vi "DataWriteTxt.vi"(0 "DataFileRef":refnum<file>, 9 "NewDataIn":dbl[](array[numeric]) format="%#_16g", 11 "error in (no error)":errorcluster) -> (4 "DataFileRef Out":refnum<file>, 10 "NewDataOut":dbl[](array[numeric]) format="%#_16g", 15 "error out":errorcluster)   [LabVIEW 2019]
doc: "Ce VI sauvegarde les données d'acquisition pour en garder une copie de sécurité qui peut être rappeller en cas de panne."
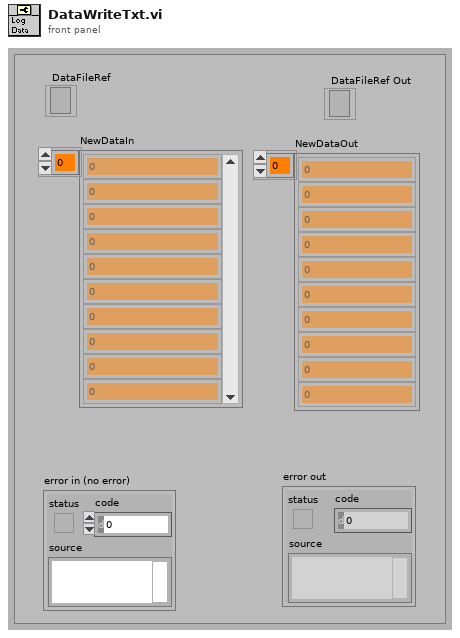
[diagram p1: front panel]
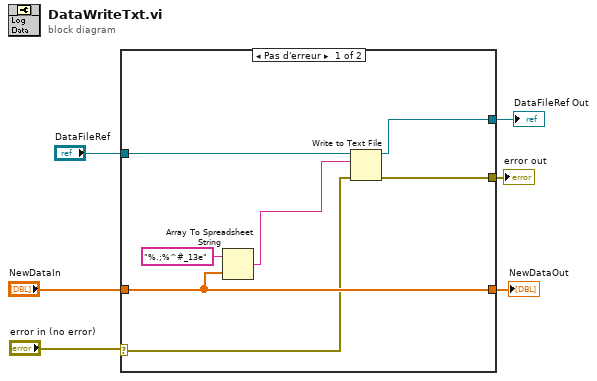
[diagram p0: block diagram]
diagram:
  n1 = case shown="Pas d'erreur" "error in (no error)" {
    selector: "error in (no error)" -> [w9 w16]
    tunnel: "NewDataIn" -> [w13 w15]
    tunnel: [w11 w16] -> w4
    tunnel: [w13 w15] -> w3
    tunnel: "DataFileRef" -> [w10 w14]
    tunnel: [w8 w14] -> w1
    frame No Error {
      n2 = Array To Spreadsheet String(array=w13, 3:"%.;%^#_13e" ("chaîne de format")) -> (spreadsheet string=w7:string)  [unwired: 1 in]
      n3 = Write to Text File(file (use dialog)=w10, text=w7, error in=w9) -> (refnum out=w8:refnum<file>, error out=w11:errorcluster)  [unwired: 1 in, 1 out]
    }
    frame Error {
    }
  }
  "NewDataOut" <- w3
  "error out" <- w4
  "DataFileRef Out" <- w1
